vi "GetAlarms.vi"(8 "error in (no error)":errorcluster) -> (0 "error out":errorcluster, 1 "found":bool, 3 "alarm rules":T1[](array[typedef]))   [LabVIEW 2017, in "GlobalConfiguration.lvlib"]
doc: "Returns information about each alarm rule the device monitors."
uses:
  <vilib>/addons/InsightCM/Utilities/GlobalConfiguration/GlobalConfiguration.lvlib
  <vilib>/addons/InsightCM/MessageBus/Base/controls/AlarmRule.ctl
  <vilib>/addons/InsightCM/MessageBus/Base/controls/AlarmTrigger.ctl
  <vilib>/addons/InsightCM/MessageBus/Base/controls/AlarmCondition.ctl
  <vilib>/addons/InsightCM/MessageBus/Base/controls/AlarmAction.ctl
  <vilib>/addons/InsightCM/MessageBus/Base/controls/KeyValuePair.ctl
  <vilib>/addons/PointValueMap/subVIs/Point_Read_variant.vi
  <vilib>/addons/PointValueMap/subVIs/Point_Write_variant.vi
  <vilib>/addons/PointValueMap/PointValueMap.lvlib
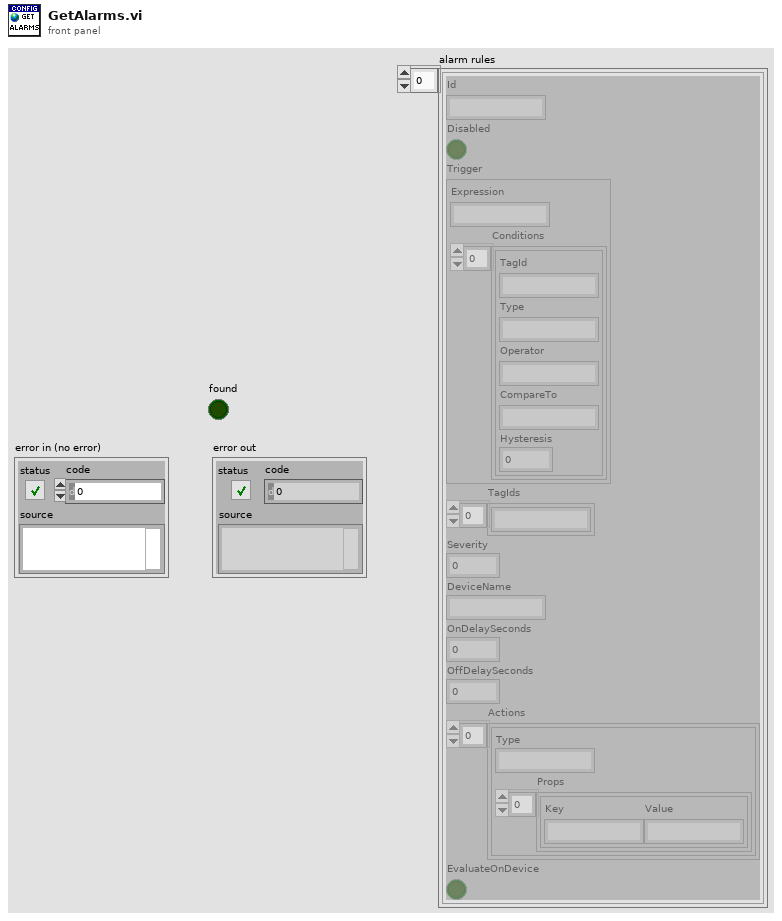
[diagram p1: front panel]
types:
  T1 = typedef "AlarmRule.ctl" = cluster{"Id":string, "Disabled":bool, "Trigger":T2, "TagIds":string[], "Severity":i32, "DeviceName":string, "OnDelaySeconds":dbl, "OffDelaySeconds":dbl, "Actions":T4[], "EvaluateOnDevice":bool}
  T2 = typedef "AlarmTrigger.ctl" = cluster{"Expression":string, "Conditions":T3[]}
  T3 = typedef "AlarmCondition.ctl" = cluster{"TagId":string, "Type":string, "Operator":string, "CompareTo":string, "Hysteresis":dbl}
  T4 = typedef "AlarmAction.ctl" = cluster{"Type":string, "Props":T5[]}
  T5 = typedef "KeyValuePair.ctl" = cluster{"Key":string, "Value":string}
  T6 = typedef "PointValueMap.lvlib/PointMap.ctl" = refnum<data-value>
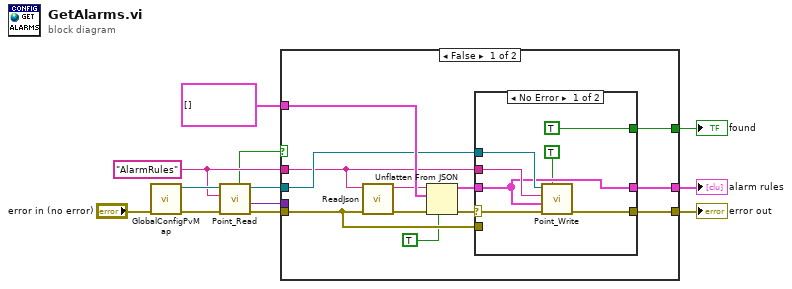
[diagram p0: block diagram]
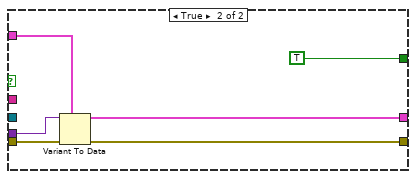
[diagram p3: hidden frame]
diagram:
  w6 = "AlarmRules" ("Name")
  n1 = call <vilib>:"GlobalConfigPvMap.vi"("error in (no error)"="error in (no error)") -> ("error out"=w11:errorcluster, "global configuration map"=w10:T6)  [unwired: 9 in]
  n2 = call-poly <vilib>:"Point_Read.vi"("Error In"=w11, "Tag"=w6, "Map"=w10) -> ("Error Out"=w2:errorcluster, "Value"=w1:variant, "Map Out"=w12:T6, "Valid?"=w3:bool)  [unwired: 3 in, 2 out]
  n3 = case shown="False" w3 {
    tunnel: [w15 w38] -> w8
    tunnel: [w16 w37] -> w5
    tunnel: [w20 TRUE] -> w4
    tunnel: w6 -> [w18 _]
    tunnel: T1[] [] ("Metrics 2") -> [w23 w35]
    tunnel: w12 -> [w19 _]
    tunnel: w2 -> [w14 w34]
    tunnel: w1 -> [_ w33]
    frame False {
      n4 = call <vilib>:"ReadJson.vi"("error in (no error)"=w14, "json object"=w18) -> ("error out"=w24:errorcluster, "json string"=w22:string)  [unwired: 8 in]
      n5 = Unflatten From JSON(JSON string=w22, type and defaults=w23, default null elements? (F)=TRUE, error in (no error)=w24) -> (value=w17:T1[], error out=w21:errorcluster)  [unwired: 3 in]
      n6 = case shown="No Error" w21 {
        selector: w21 -> [w31 _]
        tunnel: [TRUE _] -> w20
        tunnel: w19 -> [w29 _]
        tunnel: w18 -> [w28 _]
        tunnel: w17 -> [w27 _]
        tunnel: [w27 _] -> w16
        tunnel: [w26 w32] -> w15
        tunnel: w14 -> [_ w32]
        frame No Error {
          n7 = call-poly <vilib>:"Point_Write.vi"("Auto Create?"=TRUE, "Error In"=w31, "Value"=w27, "Tag"=w28, "Map"=w29) -> ("Error Out"=w26:errorcluster)  [unwired: 5 in, 1 out]
        }
        frame Error {
        }
      }
    }
    frame True {
      n8 = Variant To Data(error in=w34, type=w35, Variant=w33) -> (data=w37:T1[], error out=w38:errorcluster)
    }
  }
  "error out" <- w8
  "alarm rules" <- w5
  "found" <- w4
